vi "Create-Destroy.vi"(8 "Error In":errorcluster) -> (0 "Error Out":errorcluster)   [LabVIEW 2017, in "Tests.lvlib" / "Reader.lvlib"]
uses:
  Reader.lvlib
  <vilib>/addons/_JKI Toolkits/Caraya/classes/Test/Test.lvclass
  src/LabPack/Public/Reader/Reader.lvclass
  <vilib>/addons/_JKI Toolkits/Caraya/classes/Assert/Assert.lvclass
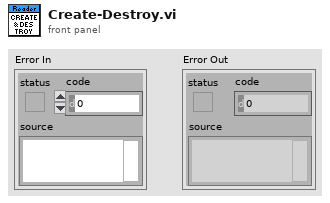
[diagram p1: front panel]
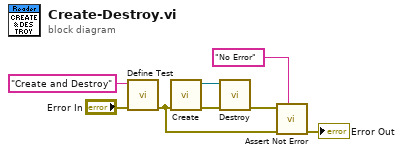
[diagram p0: block diagram]
diagram:
  n1 = call <vilib>:"Define Test.vi"("error in (no error)"="Error In", "Label (VI Title)"="Create and Destroy") -> ("error out"=w4:errorcluster)  [unwired: 9 in]
  n2 = call "Create.vi"("Error In"=w4) -> ("Error Out"=w1:errorcluster, "Reader"=w2:refnum<class "Reader.lvclass">)  [unwired: 9 in]
  n3 = call "Destroy.vi"("Error In"=w1, "Reader"=w2) -> ("Error Out"=w6:errorcluster)  [unwired: 9 in]
  n4 = call <vilib>:"Assert Not Error.vi"("Label"="No Error", "error in (no error)"=w4, "Not Error?"=w6) -> ("error out"=→"Error Out":errorcluster)  [unwired: 8 in]
